vi "Gray's Mod Motor Controler.vi"() -> ()   [LabVIEW 2009]
uses:
  <vilib>/eio/EIONode/EIONode.xnode
  <vilib>/rvi/eio/nirviEIOImplementation/nirviEIOImplementation.xnode
  <vilib>/rvi/eio/common/nirviEmuTemplateMethod_noerrors.vi
  <vilib>/rvi/eio/common/nirviEmuClasses.ctl
  <vilib>/Platform/TimedLoop/XDataNode/XDataNode.xnode
  <vilib>/Platform/TimedLoop/XDataNode/loadlvalarms.vi
  <vilib>/Platform/TimedLoop/XDataNode/timing_clust.ctl
  <vilib>/Platform/TimedLoop/XDataNode/nitl_modes.ctl
  <vilib>/Platform/TimedLoop/XDataNode/wakeup.ctl
  <vilib>/Platform/TimedLoop/XDataNode/XDNodeRunTimeDep.lvlib
panel:
  in  "Steering Encoder Reset \nPosition Whole Rotations":i32
  in  "Counts per Drive Position 2":i32=205386
  in  "Drive Encoder Reset \nPosition Fractional":i32
  in  "Counts per Drive Position":i32=205386
  in  "Stop":bool=TRUE
  out "Drive Motor Speed (cpt)":fxp<+/-,20,1>
  out "Drive Encoder Delta (ticks)":u32
  in  "Drive Motor Speed Setpoint (mph)":fxp<+/-,20,7>
  in  "Drive Speed Proportional Control Feedback Gain":fxp<+/-,20,5>
  out "Drive Motor Speed (Volts)":fxp<+/-,20,5> format="%.17g"
  in  "Drive Conversion: \nmph to counts per tick":fxp<+/-,20,0>
  in  "Drive Encoder Offset":fxp<+/-,20,1>
  in  "Steering Proportional Control Feedback Gain":fxp<+/-,20,5>
  in  "Steer Motor Setpoint (degrees)":fxp<+/-,10,7>
  in  "Steering Encoder Offset from 0 counts":fxp<+/-,32,32>
  in  "Steering Conversion: degrees to ticks":fxp<+/-,32,32>
  out "Steering Motor Speed (Volts)":fxp<+/-,20,5> format="%.17g"
  out "Steering Position":i32
  out "Steering Encoder Index":i32
  out "Steering Encoder Raw":i32
  in  "Steering Encoder Reset":bool
  in  "Steering Encoder Reset \nPositions Fractional":i32
  out "Steering clock ticks/encoder count":u32
  in  "Drive Encoder Reset":bool
  in  "Drive Encoder Reset \nPosition Whole Rotations":i32
  out "Drive Encoder Index":i32
  out "Drive Position":i32
  # "Drive Motor Control"
  # "Steering Motor Control"
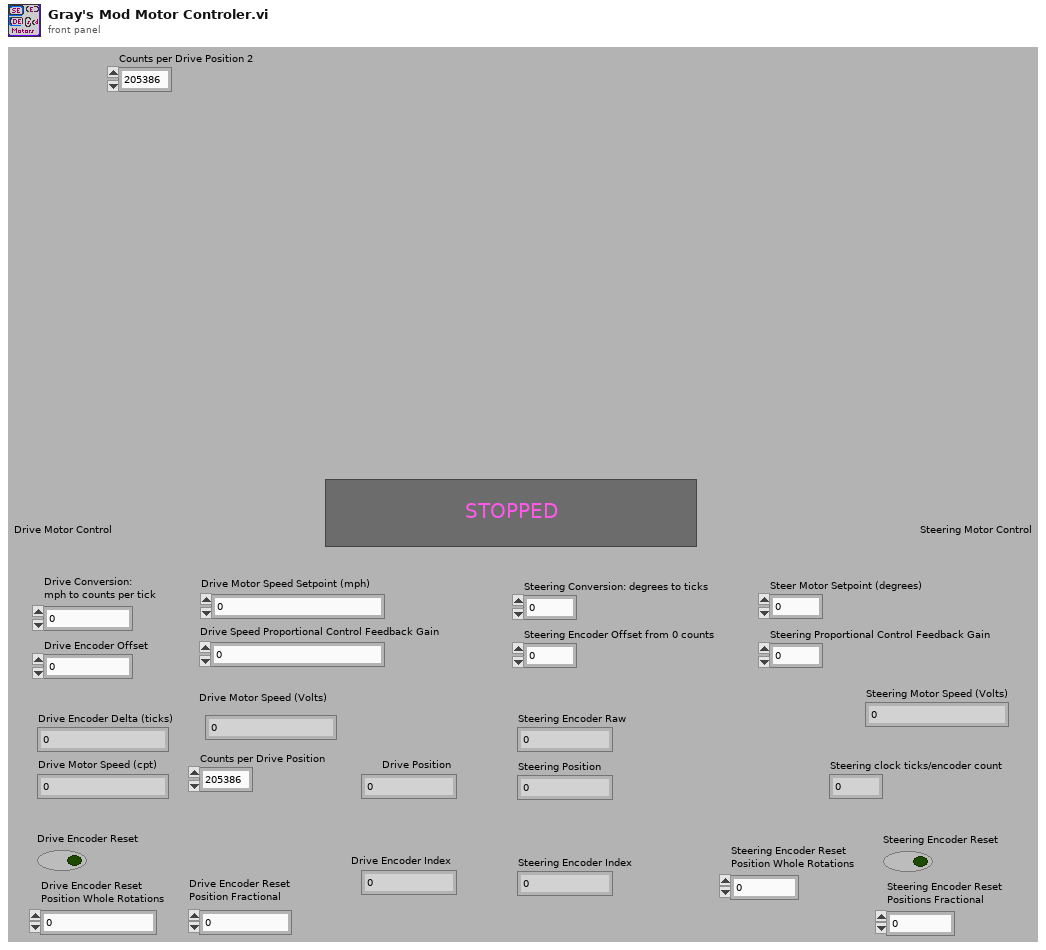
[diagram p1: front panel]
types:
  T1 = typedef "XDNodeRunTimeDep.lvlib/timing_clust.ctl" = cluster{"Expected End [f-1]":u64, "Actual End [f-1]":u64, "Finished Late? [f-1]":bool, "Expected End [i-1]":u64, "Actual End [i-1]":u64, "Finished Late? [i-1]":bool, "Expected Start [i]":u64, "Actual Start [i]":u64, "Expected Start [f]":u64, "Actual Start [f]":u64, "Source Name":string, "Structure Name":string, "Period":i64, "Deadline":i64, "Offset":i64, "Start":i64, "Priority":i32, "Timeout":i32, "Mode":T2, "Wakeup Reason":T3, "Error":errorcluster, "Source Type":string, "Secondary Source Type":string, "Global End Time":u64, "Global Start Time":u64, "Frame Duration":u64, "Iteration Duration":u64, "Assigned CPU":i32, "I/O Scan Engine Mode":u32}
  T2 = typedef "XDNodeRunTimeDep.lvlib/nitl_modes.ctl" = enum32{"No Change", "Process missed periods, maintain original phase", "Discard missed periods, maintain original phase", "Process missed periods, ignore original phase", "Discard missed periods, ignore original phase"}
  T3 = typedef "XDNodeRunTimeDep.lvlib/wakeup.ctl" = enum32{"Normal", "Aborted", "Asynchronous wakeup", "Timing source error", "Timed loop error", "Timeout"}
  T4 = typedef "nirviEmuClasses.ctl" = enum16{"IO Read", "IO Write", "Method", "Property Read", "Property Write"}
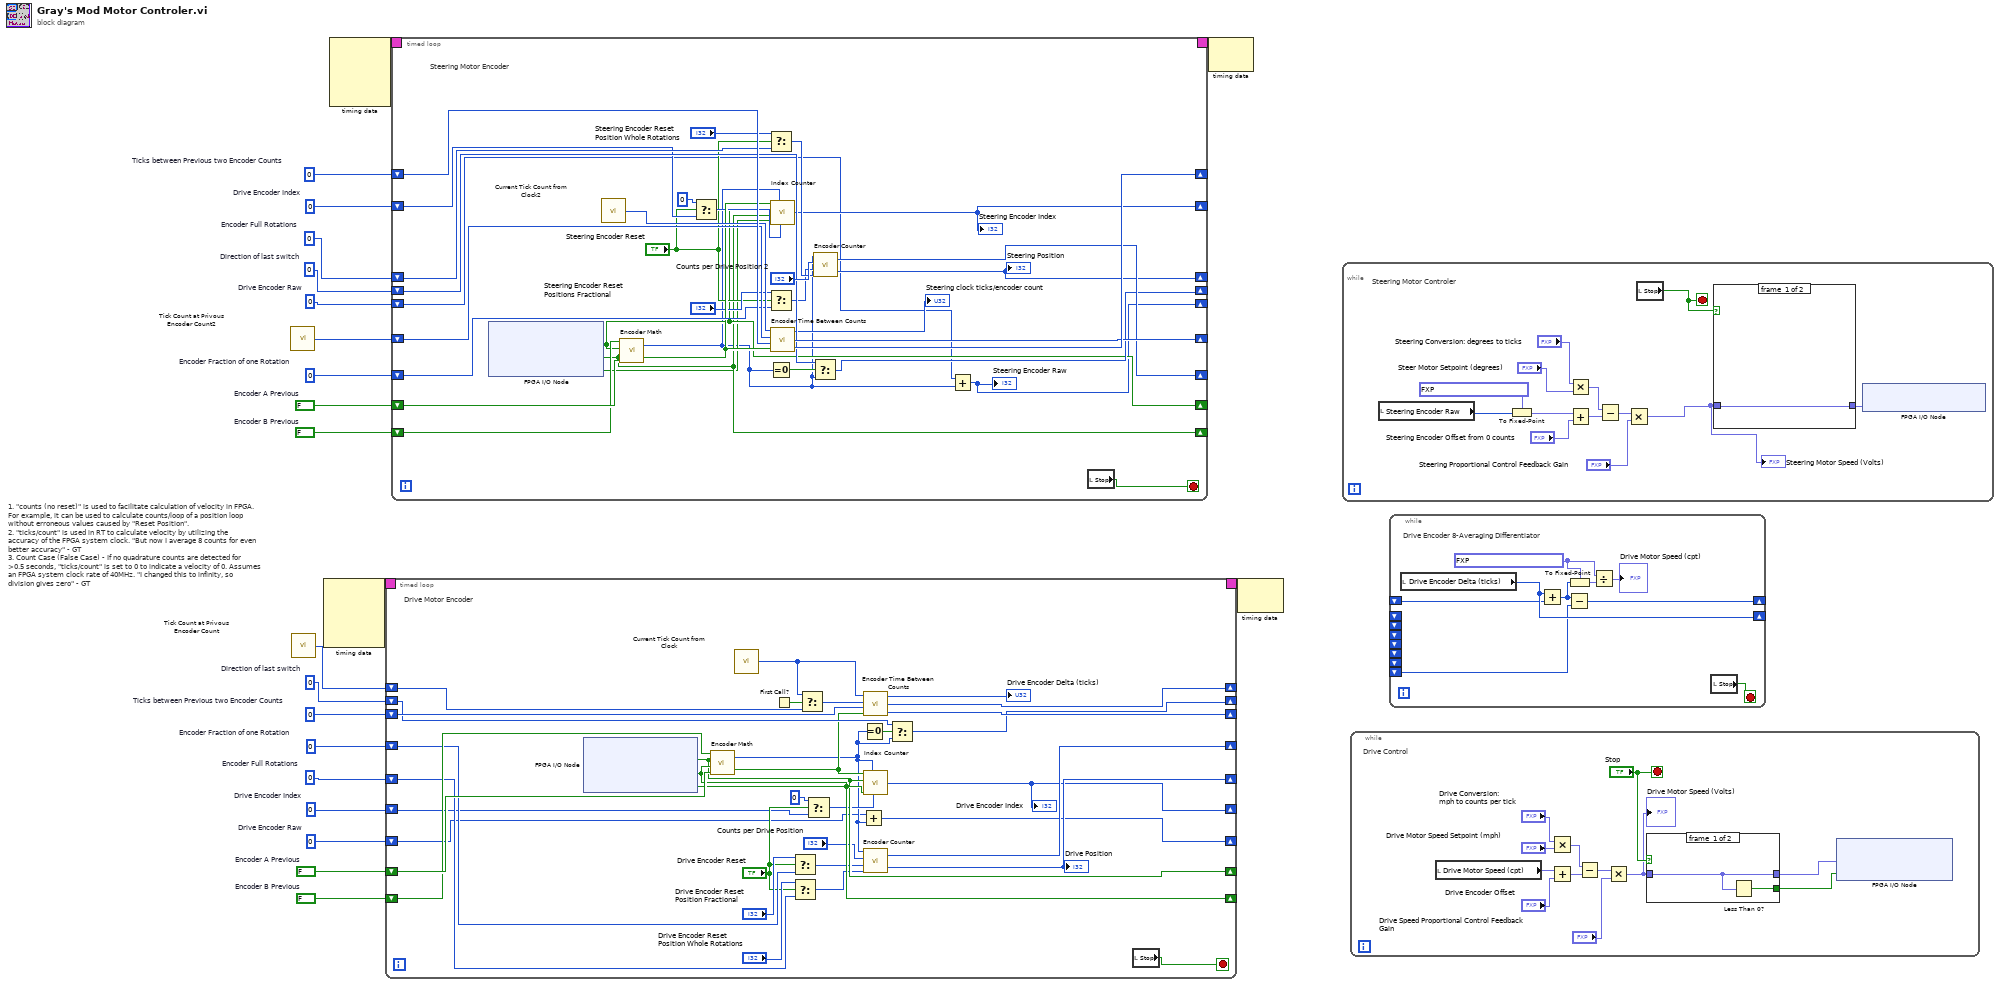
[diagram p0: block diagram]
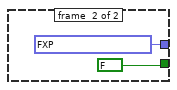
[diagram p2: hidden frame]
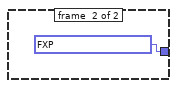
[diagram p3: hidden frame]
diagram:
  w9 = 0  # Direction of last switch
  w7 = FALSE  # Encoder B Previous
  w6 = FALSE  # Encoder A Previous
  w1 = 0  # Drive Encoder Raw
  w5 = u32 0  # Ticks between Previous two Encoder Counts
  w2 = 0  # Drive Encoder Index
  w4 = 0  # Encoder Fraction of one Rotation
  w3 = 0  # Encoder Full Rotations
  w12 = 0  # Direction of last switch
  w14 = FALSE  # Encoder B Previous
  w15 = FALSE  # Encoder A Previous
  w20 = 0  # Drive Encoder Raw
  w16 = u32 0  # Ticks between Previous two Encoder Counts
  w19 = 0  # Drive Encoder Index
  w17 = 0  # Encoder Fraction of one Rotation
  w18 = 0  # Encoder Full Rotations
  # "1. \"counts (no reset)\" is used to facilitate calculation of velocity in FPGA.\nFor example, it can be used to calculate counts/loop of a position loop\nwithout erroneous values caused by \"Reset Position\". \n2. \"ticks/count\" is used in RT to calculate velocity by utilizing the\naccuracy of the FPGA system clock. \"But now I average 8 counts for even\nbetter accuracy\" - GT\n3. Count Case (False Case) - If no quadrature counts are detected for\n>0.5 seconds, \"ticks/count\" is set to 0 to indicate a velocity of 0. Assumes\nan FPGA system clock rate of 40MHz. \"I changed this to infinity, so\ndivision gives zero\" - GT"
  n1 = call "Tick Count at Privous Encoder Count2"() -> ("Tick Count(Ticks)"=w8:u32)
  n2 = call "Tick Count at Privous Encoder Count"() -> ("Tick Count(Ticks)"=w13:u32)
  n3 = node-c288() -> (w22:T1)  [unwired: 4 in]
  n4 = node-c288() -> (w11:T1)  [unwired: 4 in]
  n5 = timed-loop {
    shift-right: [w53] -> _
    shift-left: w15 -> [w57]
    shift-right: [w55] -> _
    shift-left: w14 -> [w52]
    shift-right: [w34] -> _
    shift-left: w19 -> [w31]
    shift-right: [w49] -> _
    shift-left: w13 -> [w24]
    shift-right: [w50] -> _
    shift-left: w16 -> [w51]
    timing: w22 -> [_]
    timing-out: [_] -> w21
    shift-right: [w27] -> _
    shift-left: w20 -> [w28]
    shift-right: [w46] -> _
    shift-left: w18 -> [w41]
    shift-right: [w47] -> _
    shift-left: w17 -> [w37]
    shift-right: [w43] -> _
    shift-left: w12 -> [w44]
    stop <- w54 stop-if-true
    # "Drive Motor Encoder"
    n6 = xnode "FPGA I/O Node"() -> ("Drive Encoder A"=w53:bool, "Drive Encoder B"=w55:bool, "Drive Encoder Index"=w56:bool)  [unwired: 3 in, 3 out]
    n7 = call "Encoder Math.vi"("Encoder A_old"=w57, "Encoder B_old"=w55, "Encoder A_new"=w53, "Encoder B_new"=w52) -> ("The Encoder Changed"=w35:bool, "Change in Encoder Value"=w29:i32)
    n8 = call "Current Tick Count from Clock"() -> ("Tick Count(Ticks)"=w25:u32)
    n9 = First Call?() -> (First Call?: T/F=w26:bool)
    n10 = Select(t="Drive Encoder Reset \nPosition Fractional", s="Drive Encoder Reset", f=w37) -> (s? t:f=w36:i32)
    n11 = Select(t="Drive Encoder Reset \nPosition Whole Rotations", s="Drive Encoder Reset", f=w41) -> (s? t:f=w40:i32)
    n12 = Select(t=w25, s=w26, f=w24) -> (s? t:f=w23:u32)
    n13 = Select(t=0, s="Drive Encoder Reset", f=w31) -> (s? t:f=w30:i32)
    n14 = Add(x=w28, y=w29) -> (x+y=w27:i32)
    n15 = Equal To 0?(x=w29) -> (x = 0?=w45:bool)
    n16 = call "Encoder Time Between Counts.vi"("The Encoder Changed"=w35, "Ticks between Previous two Encoder Counts (n-1)"=w51, "Tick Count at Previous Encoder Count (n-1)"=w23, "Current Tick Count"=w25) -> ("Ticks between Previous two Encoder Counts (n)"=w50:u32, "Tick Count at Previous Encoder Count (n)"=w49:u32, "Encoder Delta (ticks)"=→"Drive Encoder Delta (ticks)":u32)
    n17 = call "Index Counter.vi"("Encoder Index (n-1)"=w30, "Change in Encoder Value"=w29, "Encoder Index Pin"=w56, "Encoder B Pin"=w55, "Encoder A Pin"=w53, "The Encoder Changed"=w35) -> ("Encoder Index (n)"=w34:i32)
    "Drive Encoder Index" <- w34
    n18 = call "Encoder Counter.vi"("Encoder Full Rotations (n-1)"=w40, "Encoder Fraction of one Rotation (n-1)"=w36, "Counts per Rotation"="Counts per Drive Position", "Change in Encoder Value"=w29) -> ("Encoder Full Rotations (n)"=w46:i32, "Encoder Fraction of one Rotation (n)"=w47:i32)
    "Drive Position" <- w46
    n19 = Select(t=w44, s=w45, f=w29) -> (s? t:f=w43:i32)
    n20 = local read "Stop"() -> (w54:bool)
  }
  n21 = timed-loop {
    shift-right: [w122] -> _
    shift-left: w6 -> [w149]
    shift-right: [w121] -> _
    shift-left: w7 -> [w147]
    shift-right: [w123] -> _
    shift-left: w2 -> [w130]
    shift-right: [w142] -> _
    shift-left: w8 -> [w143]
    shift-right: [w145] -> _
    shift-left: w5 -> [w146]
    timing: w11 -> [_]
    timing-out: [_] -> w10
    shift-right: [w117] -> _
    shift-left: w1 -> [w118]
    shift-right: [w124] -> _
    shift-left: w3 -> [w136]
    shift-right: [w140] -> _
    shift-left: w4 -> [w134]
    shift-right: [w137] -> _
    shift-left: w9 -> [w138]
    stop <- w148 stop-if-true
    # "Steering Motor Encoder"
    n22 = xnode "FPGA I/O Node"() -> ("Drive Encoder A"=w122:bool, "Drive Encoder B"=w121:bool, "Drive Encoder Index"=w120:bool)  [unwired: 3 in, 3 out]
    n23 = call "Current Tick Count from Clock2"() -> ("Tick Count(Ticks)"=w144:u32)
    n24 = call "Encoder Math.vi"("Encoder A_old"=w149, "Encoder B_old"=w121, "Encoder A_new"=w122, "Encoder B_new"=w147) -> ("The Encoder Changed"=w132:bool, "Change in Encoder Value"=w119:i32)
    n25 = Select(t=0, s="Steering Encoder Reset", f=w130) -> (s? t:f=w129:i32)
    n26 = Select(t="Steering Encoder Reset \nPosition Whole Rotations", s="Steering Encoder Reset", f=w136) -> (s? t:f=w135:i32)
    n27 = Select(t="Steering Encoder Reset \nPositions Fractional", s="Steering Encoder Reset", f=w134) -> (s? t:f=w133:i32)
    n28 = Equal To 0?(x=w119) -> (x = 0?=w139:bool)
    n29 = call "Index Counter.vi"("Encoder Index (n-1)"=w129, "Change in Encoder Value"=w119, "Encoder Index Pin"=w120, "Encoder B Pin"=w121, "Encoder A Pin"=w122, "The Encoder Changed"=w132) -> ("Encoder Index (n)"=w123:i32)
    "Steering Encoder Index" <- w123
    n30 = call "Encoder Time Between Counts.vi"("The Encoder Changed"=w132, "Ticks between Previous two Encoder Counts (n-1)"=w146, "Tick Count at Previous Encoder Count (n-1)"=w143, "Current Tick Count"=w144) -> ("Ticks between Previous two Encoder Counts (n)"=w145:u32, "Tick Count at Previous Encoder Count (n)"=w142:u32, "Encoder Delta (ticks)"=→"Steering clock ticks/encoder count":u32)
    n31 = Select(t=w138, s=w139, f=w119) -> (s? t:f=w137:i32)
    n32 = call "Encoder Counter.vi"("Encoder Full Rotations (n-1)"=w135, "Encoder Fraction of one Rotation (n-1)"=w133, "Counts per Rotation"="Counts per Drive Position 2", "Change in Encoder Value"=w119) -> ("Encoder Full Rotations (n)"=w124:i32, "Encoder Fraction of one Rotation (n)"=w140:i32)
    "Steering Position" <- w124
    n33 = Add(x=w118, y=w119) -> (x+y=w117:i32)
    "Steering Encoder Raw" <- w117
    n34 = local read "Stop"() -> (w148:bool)
  }
  n35 = node-c288(w10) -> ()  [unwired: 1 out]
  n36 = node-c288(w21) -> ()  [unwired: 1 out]
  n37 = while {
    stop <- w217 stop-if-true
    # "Steering Motor Controler"
    n38 = local read "Steering Encoder Raw"() -> (w212:i32)
    n39 = To Fixed-Point(fixed-point type=fxp<+/-,32,32> 0.0, number=w212) -> (fixed-point=w211:fxp<+/-,32,32>)
    n40 = Multiply(x="Steering Conversion: degrees to ticks", y="Steer Motor Setpoint (degrees)") -> (x*y=w220:fxp<+/-,42,39>)
    n41 = Add(x=w211, y="Steering Encoder Offset from 0 counts") -> (x+y=w219:fxp<+/-,33,33>)
    n42 = Subtract(x=w220, y=w219) -> (x-y=w221:fxp<+/-,42,39>)
    n43 = Multiply(x=w221, y="Steering Proportional Control Feedback Gain") -> (x*y=w209:fxp<+/-,20,5>)
    "Steering Motor Speed (Volts)" <- w209
    n44 = local read "Stop"() -> (w217:bool)
    n45 = case shown="False" w217 {
      tunnel: w209 -> [w222 _]
      tunnel: [w222 fxp<+/-,20,5> 0.0] -> w218
      frame #0 {
      }
      frame #1 {
      }
    }
    n46 = xnode "FPGA I/O Node"("Steering Motor Speed"=w218) -> ()  [unwired: 1 in, 1 out]
  }
  n47 = while {
    stop <- "Stop" stop-if-true
    # "Drive Control"
    n48 = local read "Drive Motor Speed (cpt)"() -> (w244:fxp<+/-,20,1>)
    n49 = Multiply(x="Drive Conversion: \nmph to counts per tick", y="Drive Motor Speed Setpoint (mph)") -> (x*y=w245:fxp<+/-,20,5>)
    n50 = Add(x=w244, y="Drive Encoder Offset") -> (x+y=w243:fxp<+/-,20,5>)
    n51 = Subtract(x=w245, y=w243) -> (x-y=w246:fxp<+/-,20,5>)
    n52 = Multiply(x=w246, y="Drive Speed Proportional Control Feedback Gain") -> (x*y=w236:fxp<+/-,20,5>)
    "Drive Motor Speed (Volts)" <- w236
    n53 = case shown="True" "Stop" {
      tunnel: w236 -> [w270 _]
      tunnel: [w270 fxp<+/-,20,5> 0.0] -> w242
      tunnel: [w269 FALSE] -> w235
      frame #0 {
        n54 = Less Than 0?(x=w270) -> (x < 0?=w269:bool)
      }
      frame #1 {
      }
    }
    n55 = xnode "FPGA I/O Node"("Drive Motor Speed"=w242, "Drive Motor Reverse"=w235) -> ()  [unwired: 2 in, 2 out]
  }
  n56 = while {
    shift-right: [w276] -> _
    shift-left: _ -> [w275]
    shift-right: [w278] -> _
    shift-left: _ -> [_]
    shift-left: _ -> [_]
    shift-left: _ -> [_]
    shift-left: _ -> [_]
    shift-left: _ -> [_]
    shift-left: _ -> [_]
    shift-left: _ -> [w274]
    stop <- w279 stop-if-true
    w280 = fxp<+/-,32,32> 8.0 ("fixed-point type")
    # "Drive Encoder 8-Averaging Differentiator"
    n57 = local read "Drive Encoder Delta (ticks)"() -> (w278:u32)
    n58 = Add(x=w278, y=w275) -> (x+y=w277:u32)
    n59 = Subtract(x=w277, y=w274) -> (x-y=w276:u32)
    n60 = To Fixed-Point(fixed-point type=w280, number=w277) -> (fixed-point=w281:fxp<+/-,32,32>)
    n61 = Divide(x=w280, y=w281) -> (x/y=→"Drive Motor Speed (cpt)":fxp<+/-,20,9>)
    n62 = local read "Stop"() -> (w279:bool)
  }
